vi "InitTest.vi"() -> ()   [LabVIEW 2010]
uses:
  MakeFullImmitationStepDLL.dll
panel:
  in  "Numeric":i8
  out "algOutputPorts 2":i8[](array[numeric])
  out "algInputPorts 2":i8[](array[numeric])
  in  "algOutputPorts":i8[](array[numeric])
  in  "algInputPorts":i8[](array[numeric])
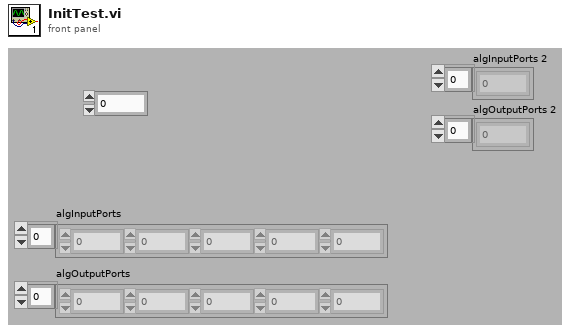
[diagram p1: front panel]
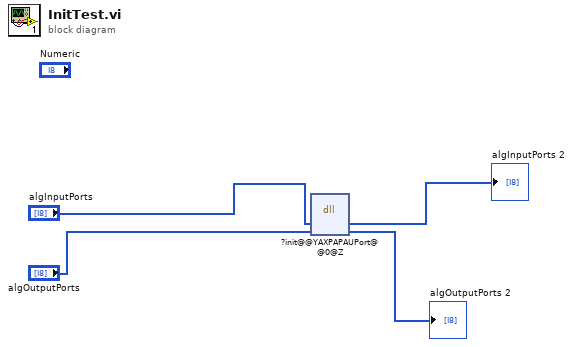
[diagram p0: block diagram]
diagram:
  n1 = dll-call lib="D:/Liakh Tanya/Dissertation/Complex/DLL-s/MakeFullImmitationStepDLL/Release/MakeFullImmitationStepDLL.dll" fn="?init@@YAXPAPAUPort@@0@Z" label="Init"("algInputPorts"="algInputPorts", "algOutputPorts"="algOutputPorts") -> ("algInputPorts"=→"algInputPorts 2":i8[], "algOutputPorts"=→"algOutputPorts 2":i8[])  [unwired: 4 in, 2 out]
